vi "update_weights.vi"(6 "Back Output":dbl[](array[numeric]), 9 "Delta":dbl[](array[numeric]), 10 "Learning Parameter":dbl, 11 "Weights":dbl[][](array[numeric])) -> (3 "Updated Weights":dbl[][](array[numeric]))   [LabVIEW 2018]
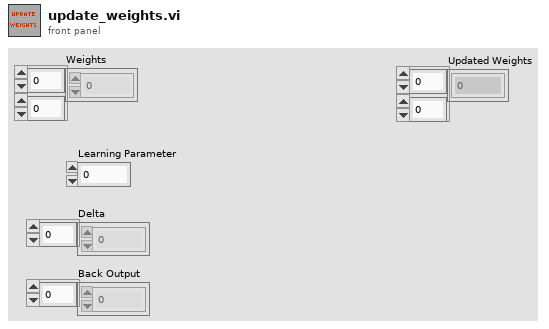
[diagram p1: front panel]
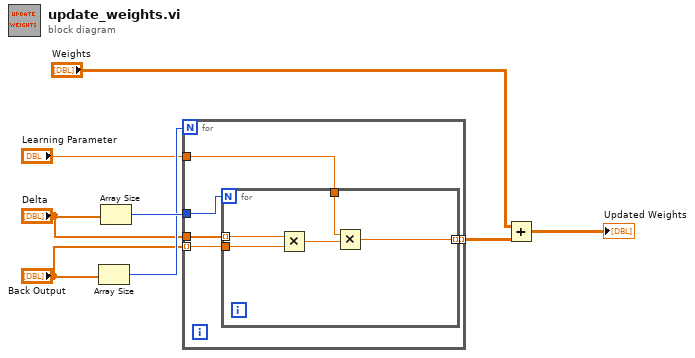
[diagram p0: block diagram]
diagram:
  n1 = Array Size(array="Back Output") -> (size(s)=w7:i32)
  n2 = Array Size(array="Delta") -> (size(s)=w8:i32)
  n3 = for {
    N: w7 -> [_]
    tunnel: w8 -> [w13]
    tunnel: "Delta" -> [w12]
    tunnel: "Back Output" -> [w11] mode=indexing
    tunnel: "Learning Parameter" -> [w10]
    tunnel: [w9] -> w3 mode=indexing
    n4 = for {
      N: w13 -> [_]
      tunnel: w12 -> [w18] mode=indexing
      tunnel: w11 -> [w17]
      tunnel: w10 -> [w16]
      tunnel: [w14] -> w9 mode=indexing
      n5 = Multiply(x=w18, y=w17) -> (x*y=w15:dbl)
      n6 = Multiply(x=w16, y=w15) -> (x*y=w14:dbl)
    }
  }
  n7 = Add(x="Weights", y=w3) -> (x+y=→"Updated Weights":dbl[][])
